vi "Excel Open File.vi"(0 "TemplatePath":path, 7 "DataFilePath":path, 11 "Error In":errorcluster) -> (4 "Excel Ref Out":refnum<k7>, 6 "WorkbookS Ref Out":refnum<k7>, 8 "Workbook Ref Out":refnum<k7>, 10 "Sheets Ref Out":refnum<k7>, 15 "Error Out":errorcluster)   [LabVIEW 2013]
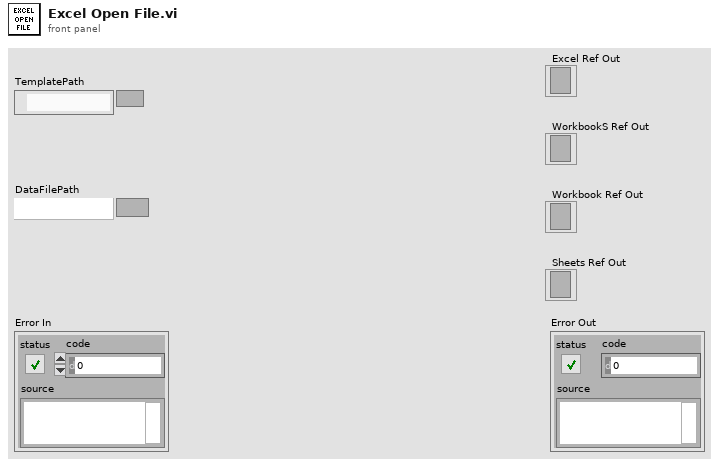
[diagram p1: front panel]
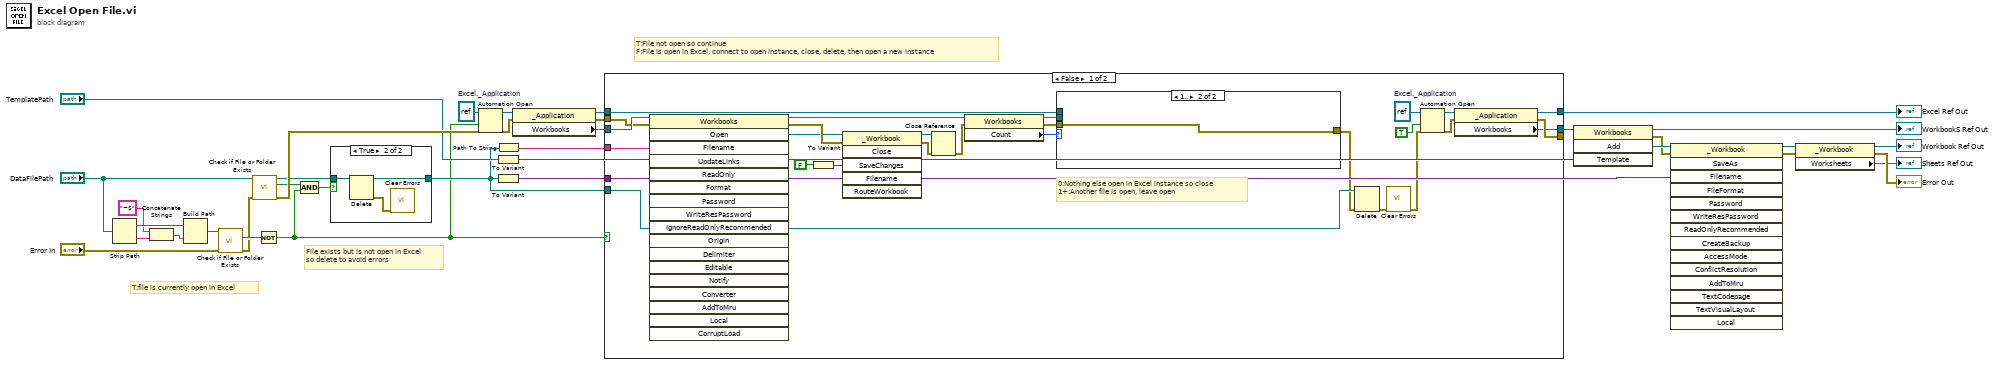
[diagram p0: block diagram]
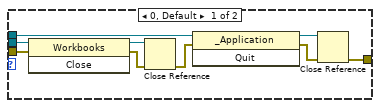
[diagram p2: hidden frame]
diagram:
  w28 = refnum<k7> refnum  # Excel._Application
  # "T:File not open so continue\nF:File is open in Excel, connect to open instance, close, delete, then open a new instance"
  # "File exists but is not open in Excel\nso delete to avoid errors"
  # "T:file is currently open in Excel"
  n1 = Strip Path(path="DataFilePath") -> (stripped path=w33:path, name=w32:string)
  n2 = Concatenate Strings("~$" ("string"), w32) -> (w30:string)
  n3 = Build Path(base path=w33, name or relative path=w30) -> (appended path=w29:path)
  n4 = call <vilib>:"Check if File or Folder Exists.vi"("error in (no error)"="Error In", "path"=w29) -> ("error out"=w24:errorcluster, "file or folder exists?"=w34:bool)  [unwired: 7 in, 1 out]
  n5 = call <vilib>:"Check if File or Folder Exists.vi"("error in (no error)"=w24, "path"="DataFilePath") -> ("error out"=w23:errorcluster, "file or folder exists?"=w10:bool)  [unwired: 7 in, 1 out]
  n6 = Not(x=w34) -> (.not. x?=w9:bool)
  n7 = And(x=w10, y=w9) -> (x .and. y?=w8:bool)
  n8 = case shown="True" w8 {
    tunnel: "DataFilePath" -> [w35 w38]
    tunnel: [w35 w37] -> w11
    frame False {
    }
    frame True {
      n9 = Delete(path (use dialog)=w38) -> (deleted path=w37:path, error out=w36:errorcluster)  [unwired: 4 in, 1 out]
      n10 = call <vilib>:"Clear Errors.vi"("error in (no error)"=w36) -> ()  [unwired: 6 in, 1 out]
    }
  }
  n11 = Automation Open(error in (no error)=w23, Automation Refnum=w28, 9:w9) -> (Automation Refnum=w26:refnum<k7>, error out=w27:errorcluster)  [unwired: 1 in]
  n12 = Path To String(path=w11) -> (string=w15:string)
  n13 = To Variant(anything="TemplatePath") -> (Variant=w16:variant)
  n14 = To Variant(anything=w11) -> (Variant=w3:variant)
  n15 = property class="_Application"(reference=w26, error in=w27) -> (reference out=w19:refnum<k7>, error out=w17:errorcluster, "Workbooks"=w18:refnum<k7>)
  n16 = case shown="False" w9 {
    tunnel: w19 -> [w58 w78]
    tunnel: w18 -> [w48 w77]
    tunnel: w17 -> [w47 w76]
    tunnel: [w50 w77] -> w12
    tunnel: [w52 w76] -> _
    tunnel: [w49 w78] -> w1
    tunnel: w11 -> [w63 _]
    tunnel: w3 -> [w64 _]
    tunnel: w15 -> [w44 _]
    frame False {
      w56 = refnum<k7> refnum  # Excel._Application
      # "0:Nothing else open in Excel instance so close\n1+:Another file is open, leave open"
      n17 = invoke class="Workbooks" method="Open"(reference=w48, error in=w47, "Filename"=w44) -> (reference out=w43:refnum<k7>, error out=w46:errorcluster, "Open"=w45:refnum<k7>)  [unwired: 15 in, 15 out]
      n18 = To Variant(anything=FALSE) -> (Variant=w62:variant)
      n19 = invoke class="_Workbook" method="Close"(reference=w45, error in=w46, "SaveChanges"=w62, "Filename"=w64) -> (reference out=w59:refnum<k7>, error out=w60:errorcluster)  [unwired: 2 in, 4 out]
      n20 = Close Reference(reference=w59, error in (no error)=w60) -> (error out=w42:errorcluster)
      n21 = property class="Workbooks"(reference=w43, error in=w42) -> (reference out=w41:refnum<k7>, error out=w40:errorcluster, "Count"=w39:i32)
      n22 = case shown="1.." w39 {
        tunnel: w58 -> [w73 _]
        tunnel: [w74 w75] -> w57
        tunnel: w41 -> [w69 _]
        tunnel: w40 -> [w68 w75]
        frame 0, Default {
          n23 = invoke class="Workbooks" method="Close"(reference=w69, error in=w68) -> (reference out=w67:refnum<k7>, error out=w66:errorcluster)  [unwired: 1 in, 1 out]
          n24 = Close Reference(reference=w67, error in (no error)=w66) -> (error out=w71:errorcluster)
          n25 = invoke class="_Application" method="Quit"(reference=w73, error in=w71) -> (reference out=w72:refnum<k7>, error out=w70:errorcluster)  [unwired: 1 in, 1 out]
          n26 = Close Reference(reference=w72, error in (no error)=w70) -> (error out=w74:errorcluster)
        }
        frame 1.. {
        }
      }
      n27 = Delete(path (use dialog)=w63, error in=w57) -> (error out=w65:errorcluster)  [unwired: 3 in, 2 out]
      n28 = call <vilib>:"Clear Errors.vi"("error in (no error)"=w65) -> ("error out"=w53:errorcluster)  [unwired: 6 in]
      n29 = Automation Open(error in (no error)=w53, Automation Refnum=w56, 9:TRUE ("open new instance (false)")) -> (Automation Refnum=w54:refnum<k7>, error out=w55:errorcluster)  [unwired: 1 in]
      n30 = property class="_Application"(reference=w54, error in=w55) -> (reference out=w49:refnum<k7>, error out=w52:errorcluster, "Workbooks"=w50:refnum<k7>)
    }
    frame True {
    }
  }
  "Excel Ref Out" <- w1
  n31 = invoke class="Workbooks" method="Add"(reference=w12, "Template"=w16) -> (reference out=→"WorkbookS Ref Out":refnum<k7>, error out=w6:errorcluster, "Add"=w7:refnum<k7>)  [unwired: 2 in, 1 out]
  n32 = invoke class="_Workbook" method="SaveAs"(reference=w7, error in=w6, "Filename"=w3) -> (reference out=w4:refnum<k7>, error out=w5:errorcluster)  [unwired: 12 in, 13 out]
  n33 = property class="_Workbook"(reference=w4, error in=w5) -> (reference out=→"Workbook Ref Out":refnum<k7>, error out=→"Error Out":errorcluster, "Worksheets"=→"Sheets Ref Out":refnum<k7>)
